vi "Asylum_Driver_XYVoltageToMeters.vi"(8 "error in (no error)":errorcluster, 9 "Y Voltage":dbl, 10 "X Voltage":dbl, 11 "Application":refnum<k7>) -> (0 "error out":errorcluster, 1 "Y Meters":dbl, 2 "X Meters":dbl, 3 "Application":refnum<k7>)   [LabVIEW 2020]
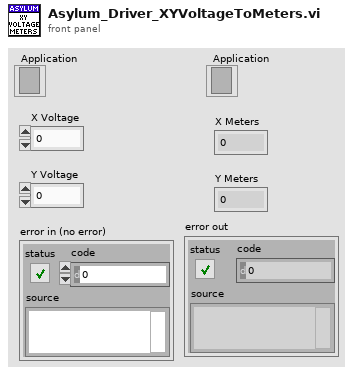
[diagram p1: front panel]
types:
  T1 = cluster{"XLVDT Sens":dbl, "YLVDT Sens":dbl, "XLVDT Offset":dbl, "YLVDT Offset":dbl}
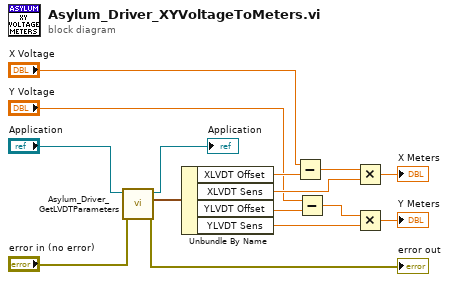
[diagram p0: block diagram]
diagram:
  n1 = call "Asylum_Driver_GetLVDTParameters.vi"("error in (no error)"="error in (no error)", "Application"="Application") -> ("error out"=→"error out":errorcluster, "LVDT Parameters"=w7:T1, "Application"=→"Application":refnum<k7>)  [unwired: 7 in]
  n2 = Unbundle By Name(w7) -> ("XLVDT Offset"=w8:dbl, "XLVDT Sens"=w10:dbl, "YLVDT Offset"=w13:dbl, "YLVDT Sens"=w12:dbl)
  n3 = Subtract(x="X Voltage", y=w8) -> (x-y=w9:dbl)
  n4 = Subtract(x="Y Voltage", y=w13) -> (x-y=w11:dbl)
  n5 = Multiply(x=w9, y=w10) -> (x*y=→"X Meters":dbl)
  n6 = Multiply(x=w11, y=w12) -> (x*y=→"Y Meters":dbl)
